vi "POP_Monitor Events.vi"() -> ()   [LabVIEW 2016]
uses:
  Ctrls/POP_Monitor Register Data.ctl
  Ctrls/POP_Event Enum.ctl
  Ctrls/POP_Popup Operation.ctl
  <vilib>/event_ctls.llb/eventvkey.ctl
  <vilib>/Utility/miscctls.llb/LVPointTypeDef.ctl
panel:
  in  "Unregister\nAll Events":bool=TRUE
  in  "Quit":refnum<user-event>
  in  "Register":refnum<user-event>
  in  "Popup":refnum<vi>
  out "error out":errorcluster
  in  "error in (no error)":errorcluster
  in  "Debug":bool
  in  "Name":string
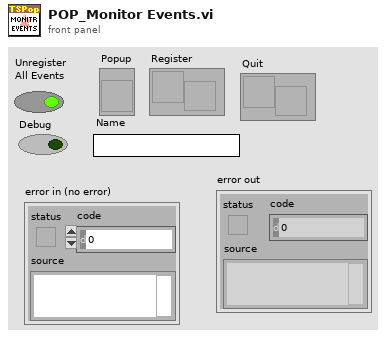
[diagram p1: front panel]
types:
  T1 = typedef "POP_Event Enum.ctl" = enum16{"Nothing", "Enter Key Accept", "Escape Key Cancel", "Mouse Outside Accept", "Mouse Outside Cancel", "Mouse Move Accept", "Mouse Move Cancel", "Mouse Leave Cancel", "Value Change Accept", "Lose Focus Cancel", "Cancel Button", "Accept Button", "Shift Ctrl Key Down"}
  T2 = typedef "eventvkey.ctl" = enum16{"ASCII", "Enter", "Return", "Shift", "Ctrl", "Alt", "Cmd", "Opt", "Caps", "NumLock", "Clear", "Break", "Up", "Down", "Left", "Right", "Insert", "Delete", "Home", "End", "PageUp", "PageDown", "Escape", "Help", "Pause", "ScrollLock", "F1", "F2", "F3", "F4", "F5", "F6", "F7", "F8", "F9", "F10", "F11", "F12", "F13", "F14", "F15", "F16", "F17", "F18", "F19", "F20", "F21", "F22", "F23", "F24", "Play", "VolumeUp", "VolumeDown", "Mute", "Two Byte Char"}
  T3 = enum32{"Bad", "Idle", "Run top level", "Running"}
  T4 = typedef "POP_Popup Operation.ctl" = enum16{"Show", "Initialize", "Close", "Popup Done", "Register a Location's Type", "Retrieve Location's Type"}
  T5 = cluster{"Shift":bool, "Ctrl":bool, "Alt":bool, "Cmd":bool, "Opt":bool}
  T6 = typedef "LVMenuShortCut.ctl" = cluster{"Include Shift Key?":bool, "Include Ctrl Key?":bool, "Shortcut Key":string}
  T7 = typedef "LVPointTypeDef.ctl" = cluster{"Horizontal":i16, "Vertical":i16}
  T8 = typedef "LVPoint32TypeDef.ctl" = cluster{"Horizontal":i32, "Vertical":i32}
  T9 = typedef "LVRectTypeDef.ctl" = cluster{"Left":i16, "Top":i16, "Right":i16, "Bottom":i16}
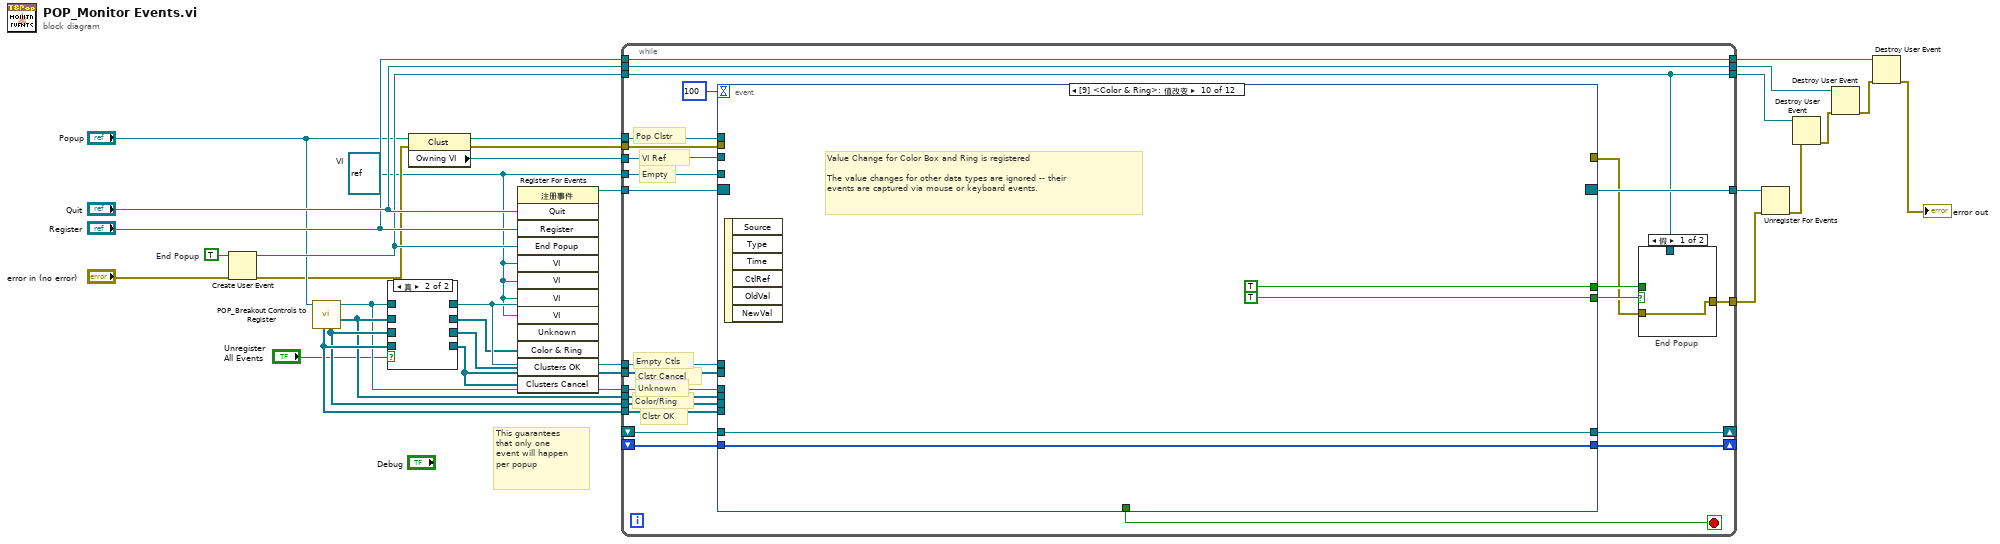
[diagram p0: block diagram]
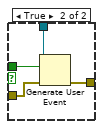
[diagram p3: hidden frame]
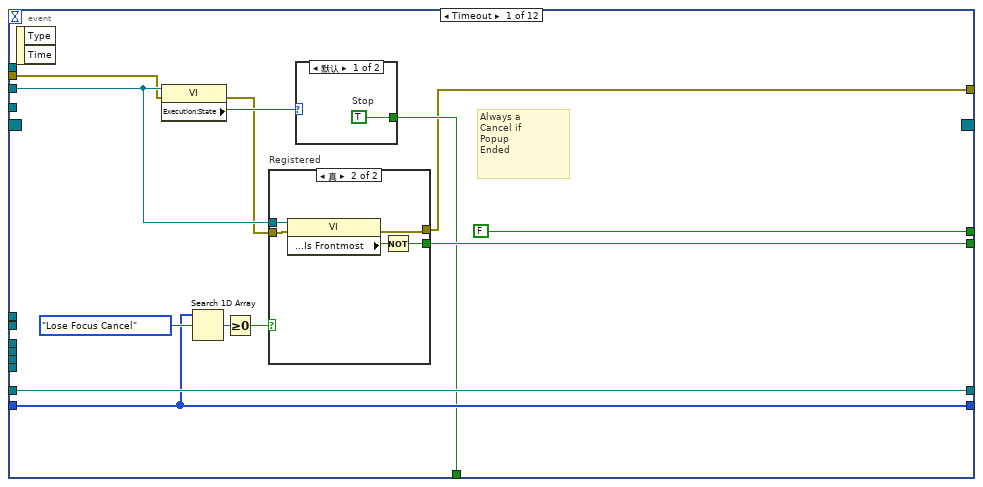
[diagram p4: hidden frame]
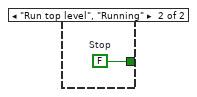
[diagram p5: hidden frame]
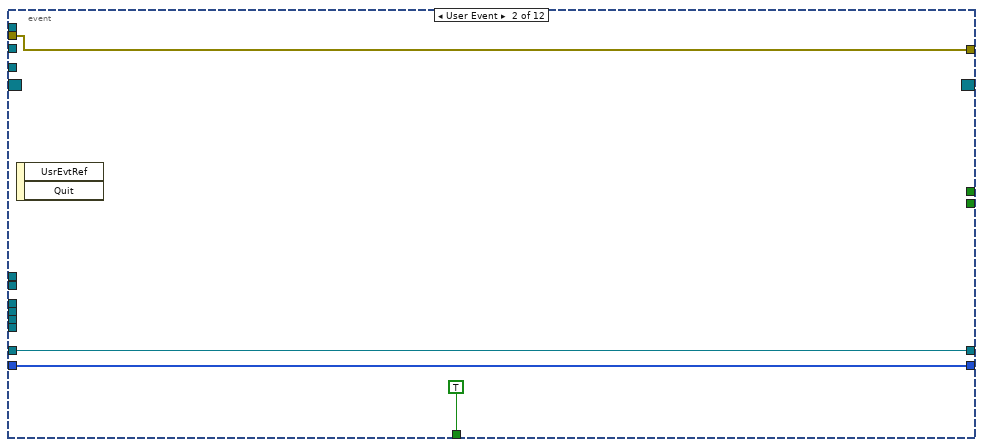
[diagram p7: hidden frame]
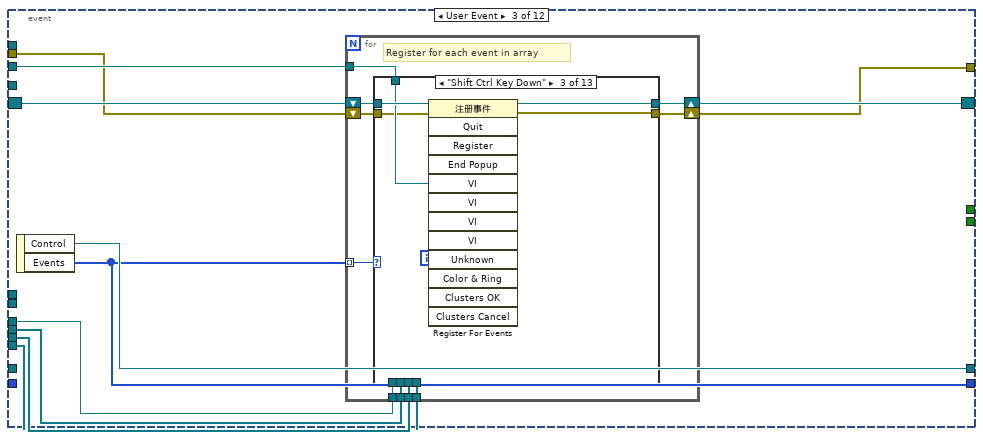
[diagram p8: hidden frame]
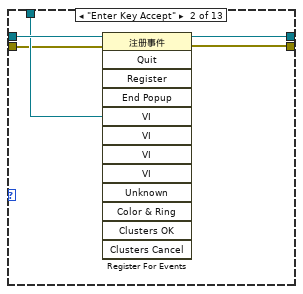
[diagram p10: hidden frame]
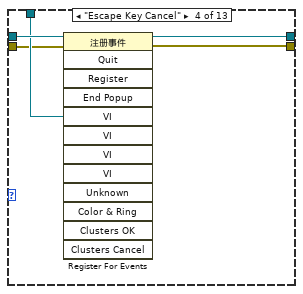
[diagram p11: hidden frame]
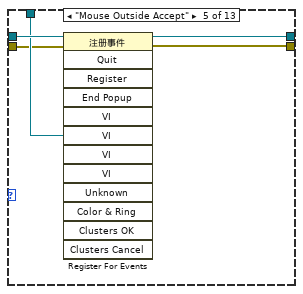
[diagram p12: hidden frame]
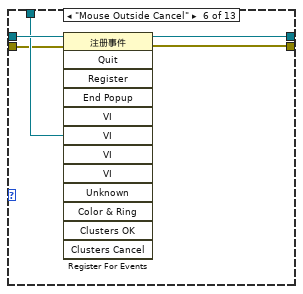
[diagram p13: hidden frame]
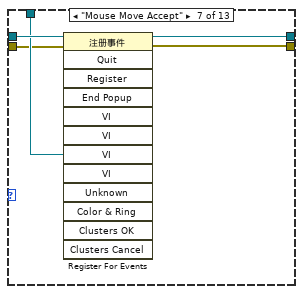
[diagram p14: hidden frame]
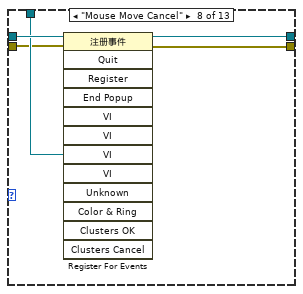
[diagram p15: hidden frame]
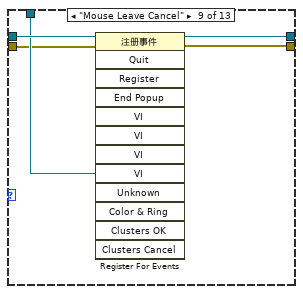
[diagram p16: hidden frame]
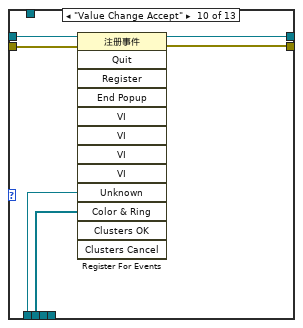
[diagram p17: hidden frame]
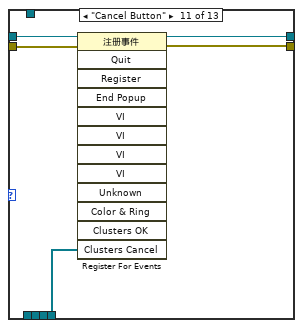
[diagram p18: hidden frame]
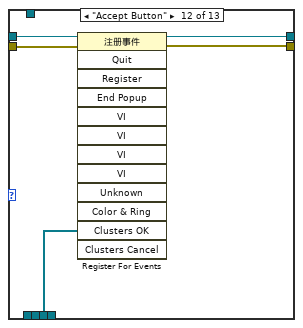
[diagram p19: hidden frame]
diagram:
  w7 = TRUE  # End Popup
  w2 = refnum<vi> refnum  # VI
  # "This guarantees\nthat only one\nevent will happen\nper popup"
  n1 = Create User Event(user event datatype=w7, error in="error in (no error)") -> (user event=w23:refnum<user-event>, error out=w3:errorcluster)
  n2 = call "POP_Breakout Controls to Register.vi"("Popup"="Popup") -> ("Color & Ring"=w19:refnum<vi>[], "Unknown"=w18:refnum<vi>, "Clusters OK"=w20:refnum<vi>[], "Clusters Cancel"=w21:refnum<vi>[])  [unwired: 7 in]
  n3 = case shown="真" "Unregister\nAll Events" {
    tunnel: [w31 _] -> w17
    tunnel: [w32 _] -> w4
    tunnel: [w33 _] -> w5
    tunnel: [w34 _] -> w16
    tunnel: w18 -> [w34 _]
    tunnel: w19 -> [w33 _]
    tunnel: w20 -> [w32 _]
    tunnel: w21 -> [w31 _]
    frame False {
    }
    frame True {
    }
  }
  n4 = property class="Clust"(reference="Popup", error in=w3) -> (reference out=w28:refnum<vi>, error out=w14:errorcluster, "Owning VI"=w1:refnum<vi>)
  n5 = register-events("Quit", "Register", w23, w2, w2, w2, w2, w16, w5, w4, w17) -> (reference out=w30:refnum<event-registration>)  [unwired: 2 in, 1 out]
  n6 = while {
    tunnel: w30 -> [w58]
    tunnel: w1 -> [w57]
    tunnel: w2 -> [w56]
    tunnel: [w55] -> w29
    tunnel: w28 -> [w54]
    tunnel: "Quit" -> [w52]
    tunnel: "Register" -> [w51]
    tunnel: [w52] -> w26
    tunnel: [w51] -> w27
    shift-right: [w50] -> _
    shift-left: _ -> [w49]
    shift-right: [w48] -> _
    shift-left: _ -> [w47]
    tunnel: w23 -> [w46]
    tunnel: [w46] -> w22
    tunnel: w21 -> [w43]
    tunnel: w20 -> [w42]
    tunnel: w19 -> [w41]
    tunnel: w18 -> [w40]
    tunnel: w17 -> [w39]
    tunnel: w16 -> [w38]
    tunnel: w14 -> [w37]
    tunnel: [w35] -> w13
    stop <- w53 stop-if-true
    # "Empty Ctls"
    # "Clstr Cancel"
    # "Clstr OK"
    # "Color/Ring"
    # "Unknown"
    # "Pop Clstr"
    # "VI Ref"
    # "Empty"
    n7 = event shown="[9] <Color & Ring>: 值改变" {
      selector: w58 -> [_ _ w99 w183 _ _ _ _ _ _ _ _]
      dyn-events: [_ _ w97 w181 _ _ _ _ _ _ _ _] -> w55
      timeout: 100 -> [_ _ _ _ _ _ _ _ _ _ _ _]
      tunnel: w57 -> [w70 _ w96 _ _ _ _ _ _ _ _ _]
      tunnel: w56 -> [_ _ _ w182 _ _ _ _ _ _ _ _]
      tunnel: w54 -> [_ _ _ _ _ w254 _ _ _ _ _ _]
      tunnel: [w68 TRUE _ _ _ _ _ _ _ _ _ _] -> w53
      tunnel: [w74 w88 w98 w185 w194 w259 w262 w270 w274 w278 w282 w286] -> w50
      tunnel: w49 -> [w74 w88 _ _ w194 w259 w262 w270 w274 w278 w282 w286]
      tunnel: [w77 w87 w100 w184 w192 w252 w266 w269 w273 w277 w281 w285] -> w48
      tunnel: w47 -> [w77 w87 _ w178 w192 w252 w266 w269 w273 w277 w281 w285]
      tunnel: [w72 _ _ _ w186 w256 TRUE TRUE TRUE TRUE TRUE TRUE] -> w45
      tunnel: [FALSE _ _ _ w187 w255 w261 FALSE FALSE TRUE TRUE FALSE] -> w44
      tunnel: w43 -> [_ _ w92 _ _ _ _ _ _ _ _ _]
      tunnel: w42 -> [_ _ w93 _ _ _ _ _ _ _ _ _]
      tunnel: w41 -> [_ _ w94 _ _ _ _ _ _ _ _ _]
      tunnel: w40 -> [_ _ w95 _ _ _ _ _ _ _ _ _]
      tunnel: w39 -> [_ _ _ w177 _ _ _ _ _ _ _ _]
      tunnel: w38 -> [_ _ _ w176 _ _ _ _ _ _ _ _]
      tunnel: w37 -> [w67 w86 w91 w175 _ w253 _ _ _ _ _ _]
      tunnel: [w65 w86 w90 w172 _ w241 _ _ _ _ _ _] -> w36
      event Timeout {
        # "Always a\nCancel if\nPopup\nEnded"
        n8 = event-data() -> ()  [unwired: 1 in, 2 out]
        n9 = property class="VI"(reference=w70, error in=w67) -> (error out=w66:errorcluster, "Execution:State"=w69:T3)  [unwired: 1 out]
        n10 = Search 1D Array(1D array=w74, element=POP_Event_Enum."Lose Focus Cancel" ("Registered Events")) -> (index of element=w76:i32)  [unwired: 1 in]
        n11 = Greater Or Equal To 0?(x=w76) -> (x >= 0?=w73:bool)
        n12 = case "Registered" shown="真" w73 {
          tunnel: w70 -> [_ w83]
          tunnel: [_ w84] -> w72
          tunnel: w66 -> [w80 w82]
          tunnel: [w80 w81] -> w65
          frame False {
          }
          frame True {
            n13 = property class="VI"(reference=w83, error in=w82) -> (error out=w81:errorcluster, "Front Panel Window:Is Frontmost"=w85:bool)  [unwired: 1 out]
            n14 = Not(x=w85) -> (.not. x?=w84:bool)
          }
        }
        n15 = case shown="默认" w69 {
          tunnel: [w78 w79] -> w68
          frame Default {
            w78 = TRUE  # Stop
          }
          frame "Run top level", "Running" {
            w79 = FALSE  # Stop
          }
        }
      }
      event User Event {
        n16 = event-data() -> ()  [unwired: 1 in, 2 out]
      }
      event User Event {
        n17 = event-data() -> ("Control"=w100:refnum<vi>, "Events"=w98:T1[])  [unwired: 1 in]
        n18 = for {
          shift-right: [w108] -> w97
          shift-left: w99 -> [w109]
          tunnel: w98 -> [w110] mode=indexing
          tunnel: w96 -> [w107]
          tunnel: w95 -> [w103]
          tunnel: w94 -> [w106]
          tunnel: w93 -> [w104]
          tunnel: w92 -> [w105]
          shift-right: [w101] -> w90
          shift-left: w91 -> [w102]
          # "Register for each event in array"
          n19 = case shown="\"Shift Ctrl Key Down\"" w110 {
            tunnel: w109 -> [w112 w117 w122 w126 w132 w137 w142 w147 w152 w158 w163 w168 w170]
            tunnel: [w112 w116 w121 w127 w131 w136 w141 w146 w151 w157 w162 w167 w170] -> w108
            tunnel: w107 -> [_ w115 w120 w125 w130 w135 w140 w145 w150 _ _ _ _]
            tunnel: w106 -> [_ _ _ _ _ _ _ _ _ w156 _ _ _]
            tunnel: w105 -> [_ _ _ _ _ _ _ _ _ _ w161 _ _]
            tunnel: w104 -> [_ _ _ _ _ _ _ _ _ _ _ w166 _]
            tunnel: w103 -> [_ _ _ _ _ _ _ _ _ w155 _ _ _]
            tunnel: w102 -> [w111 w114 w119 w124 w129 w134 w139 w144 w149 w154 w160 w165 w169]
            tunnel: [w111 w113 w118 w123 w128 w133 w138 w143 w148 w153 w159 w164 w169] -> w101
            frame "Nothing" {
              # "Nothing to register, this\nis default enum value"
            }
            frame "Enter Key Accept" {
              n20 = register-events(reference=w117, error in=w114, w115) -> (reference out=w116:refnum<event-registration>, error out=w113:errorcluster)  [unwired: 10 in]
            }
            frame "Shift Ctrl Key Down" {
              n21 = register-events(reference=w122, error in=w119, w120) -> (reference out=w121:refnum<event-registration>, error out=w118:errorcluster)  [unwired: 10 in]
            }
            frame "Escape Key Cancel" {
              n22 = register-events(reference=w126, error in=w124, w125) -> (reference out=w127:refnum<event-registration>, error out=w123:errorcluster)  [unwired: 10 in]
            }
            frame "Mouse Outside Accept" {
              n23 = register-events(reference=w132, error in=w129, w130) -> (reference out=w131:refnum<event-registration>, error out=w128:errorcluster)  [unwired: 10 in]
            }
            frame "Mouse Outside Cancel" {
              n24 = register-events(reference=w137, error in=w134, w135) -> (reference out=w136:refnum<event-registration>, error out=w133:errorcluster)  [unwired: 10 in]
            }
            frame "Mouse Move Accept" {
              n25 = register-events(reference=w142, error in=w139, w140) -> (reference out=w141:refnum<event-registration>, error out=w138:errorcluster)  [unwired: 10 in]
            }
            frame "Mouse Move Cancel" {
              n26 = register-events(reference=w147, error in=w144, w145) -> (reference out=w146:refnum<event-registration>, error out=w143:errorcluster)  [unwired: 10 in]
            }
            frame "Mouse Leave Cancel" {
              n27 = register-events(reference=w152, error in=w149, w150) -> (reference out=w151:refnum<event-registration>, error out=w148:errorcluster)  [unwired: 10 in]
            }
            frame "Value Change Accept" {
              n28 = register-events(reference=w158, error in=w154, w155, w156) -> (reference out=w157:refnum<event-registration>, error out=w153:errorcluster)  [unwired: 9 in]
            }
            frame "Cancel Button" {
              n29 = register-events(reference=w163, error in=w160, w161) -> (reference out=w162:refnum<event-registration>, error out=w159:errorcluster)  [unwired: 10 in]
            }
            frame "Accept Button" {
              n30 = register-events(reference=w168, error in=w165, w166) -> (reference out=w167:refnum<event-registration>, error out=w164:errorcluster)  [unwired: 10 in]
            }
            frame "Lose Focus Cancel" {
              # "NOOP - checked in Timeout case"
            }
          }
        }
      }
      event User Event {
        w180 = POP_Popup_Operation."Popup Done"  # Popup Operation
        w184 = refnum<vi> refnum  # Control
        w185 = T1[] [] items=["Nothing", "Enter Key Accept", "Escape Key Cancel", "Mouse Outside Accept", "Mouse Outside Cancel", "Mouse Move Accept", "Mouse Move Cancel", "Mouse Leave Cancel", "Value Change Accept", "Lose Focus Cancel", "Cancel Button", "Accept Button", "Shift Ctrl Key Down"]  # Events
        n31 = event-data() -> ("End Popup"=w179:bool)  [unwired: 1 in]
        n32 = register-events(reference=w183, error in=w175, w182, w182, w182, w182, w176, w177, w177, w177) -> (reference out=w181:refnum<event-registration>, error out=w174:errorcluster)  [unwired: 3 in]
        n33 = call "POP_FG.Popup.vi"("Popup Operation"=w180, "Name"="Name", "Error In"=w174, "Popup Accepted?"=w179) -> ("Error Out"=w173:errorcluster)  [unwired: 8 in, 3 out]
        n34 = Close Reference(reference=w178, error in (no error)=w173) -> (error out=w172:errorcluster)
      }
      event Key Down? {
        w201 = POP_Event_Enum."Escape Key Cancel"  # element
        # "Enter = Accept Popup"
        # "Registered Key Pressed"
        # "Check that key is \nRegistered and Pressed"
        # "Verify that\nkey was also\nregistered"
        # "Check if correct\nkey was pressed"
        n35 = event-data() -> ("VKey"=w190:T2, "FocusObj"=w193:refnum<vi>, "Char"=w191:i16, "PlatMods"=w189:T5)  [unwired: 1 in]
        n36 = call <vilib>:"compatReturnToEnter.vi"("VKey"=w190) -> ("VKey"=w206:T2)
        n37 = Search 1D Array(1D array=w194, element=w201) -> (index of element=w200:i32)  [unwired: 1 in]
        n38 = Search 1D Array(1D array=w194, element=POP_Event_Enum."Enter Key Accept") -> (index of element=w204:i32)  [unwired: 1 in]
        n39 = Search 1D Array(1D array=w194, element=POP_Event_Enum."Shift Ctrl Key Down" ("元素")) -> (index of element=w207:i32)  [unwired: 1 in]
        n40 = Greater Or Equal To 0?(x=w200) -> (x >= 0?=w202:bool)
        n41 = Greater Or Equal To 0?(x=w204) -> (x >= 0?=w205:bool)
        n42 = Greater Or Equal To 0?(x=w207) -> (x >= 0?=w209:bool)
        n43 = case shown="真" w209 {
          tunnel: w193 -> [_ w217]
          tunnel: w191 -> [_ w216]
          tunnel: w190 -> [_ w215]
          tunnel: w189 -> [_ w214]
          tunnel: [_ w213] -> w210
          frame False {
          }
          frame True {
            n44 = property class="GObj"(reference=w217) -> (reference out=w211:refnum<vi>, "ClassID"=w212:u32)  [unwired: 1 in, 1 out]
            n45 = case shown="27" w212 {
              tunnel: w211 -> [_ w228]
              tunnel: w216 -> [_ w221]
              tunnel: w215 -> [_ w220]
              tunnel: w214 -> [_ w219]
              tunnel: [_ w218] -> w213
              frame Default {
              }
              frame 27 {
                w227 = refnum<vi> refnum  # 字符串
                n46 = To More Specific Class(target class=w227, reference=w228) -> (specific class reference=w222:refnum<vi>)  [unwired: 1 in, 1 out]
                n47 = call "MENU_Shortcut Generate.vi"("PlatMods"=w219, "VKey"=w220, "Char"=w221) -> ("short cut"=w223:T6)  [unwired: 8 in]
                n48 = Unbundle(w223) -> ("Include Shift Key?"=w224:bool, "Include Ctrl Key?"=w225:bool, "Shortcut Key"=w226:string)
                n49 = case shown="\"True\", 默认" w226 {
                  selector: w226 -> [_ w232]
                  tunnel: w224 -> [_ w236]
                  tunnel: w225 -> [_ w235]
                  tunnel: w222 -> [_ w233]
                  tunnel: [_ TRUE] -> w218
                  frame " " {
                  }
                  frame "True", Default {
                    w237 = "" ("f")
                    # "字符串键按下"
                    n50 = Select(t="Shift+", s=w236, f=w237) -> (s? t:f=w231:string)
                    n51 = Select(t="Ctrl+", s=w235, f=w237) -> (s? t:f=w230:string)
                    n52 = Concatenate Strings(w230, w231, w232) -> (w234:string)
                    n53 = property class="Str"(reference=w233, "Value"=w234) -> ()  [unwired: 1 in, 2 out]
                  }
                }
              }
            }
          }
        }
        n54 = Equal?(x=eventvkey."Escape" ("VKey"), y=w206) -> (x = y?=w197:bool)
        n55 = Equal?(x=w206, y=eventvkey."Enter") -> (x = y?=w199:bool)
        n56 = And(x=w197, y=w202) -> (x .and. y?=w198:bool)
        n57 = And(x=w205, y=w199) -> (x .and. y?=w187:bool)
        n58 = Compound Arithmetic op=OR(w198, w187) -> (w186:bool)
        n59 = Compound Arithmetic op=OR(w186, w210) -> (w188:bool)
        n60 = event-data("Discard?"=w188) -> ()  [unwired: 1 in, 1 out]
      }
      event Mouse Down? {
        (unwired) T7 {"Horizontal"=0, "Vertical"=0} ("Pane Coordinates")
        # ">> Notes: 此处50为经验值；2014.7.30<<"
        n61 = event-data() -> ("Coords"=w240:T8)  [unwired: 1 in]
        n62 = call "POP_CtlRect.vi"("Error In"=w253, "CtlRef"=w252, "PopupRef"=w254) -> ("Error Out"=w242:errorcluster, "Panes?"=w247:bool, "Pane Refnum"=w251:refnum<vi>)  [unwired: 5 in, 1 out]
        n63 = invoke class="Pane" method="CvtPanelToPaneCoords"(reference=w251, error in=w242, "PanelCoords"=w240) -> (error out=w241:errorcluster, "PaneCoords"=w246:T7)  [unwired: 2 in, 3 out]
        n64 = Add(x=w246, y=i16 50) -> (x+y=w245:T7)
        n65 = property class="Ctl"(reference=w252) -> ("Total Bounds Rect"=w249:T9)  [unwired: 1 in, 2 out]
        n66 = Select(t=w240, s=w247, f=w245) -> (s? t:f=w244:T8)
        n67 = To Double Precision Float(number=w244) -> (double precision float=w243:cluster{"Horizontal":dbl, "Vertical":dbl})
        n68 = To Word Integer(number=w249) -> (16bit integer=w248:T9)
        n69 = call <vilib>:"PointInRect.vi"("rect"=w248, "point"=w243) -> ("pt in rect"=w257:bool)
        n70 = Not(x=w257) -> (.not. x?=w256:bool)
        n71 = Search 1D Array(1D array=w259, element=POP_Event_Enum."Mouse Outside Accept" ("Registered Events")) -> (index of element=w260:i32)  [unwired: 1 in]
        n72 = Greater Or Equal To 0?(x=w260) -> (x >= 0?=w255:bool)
        n73 = event-data("Discard?"=w256) -> ()  [unwired: 1 in, 1 out]
      }
      event Mouse Move {
        # "Used for Rings to capture when the selection doesn't change\nand for both rings and colorboxes when Escape is pressed \n(not captured with Key Press event)"
        n74 = event-data() -> ()  [unwired: 1 in, 1 out]
        n75 = Search 1D Array(1D array=w262, element=POP_Event_Enum."Mouse Move Accept" ("Registered Events")) -> (index of element=w264:i32)  [unwired: 1 in]
        n76 = Greater Or Equal To 0?(x=w264) -> (x >= 0?=w261:bool)
      }
      event Mouse Leave {
        # "Mouse Leave is (currently) always registered as a cancel.\nThis is used for Colors and Rings to capture when the Escape key is\npressed when the mouse is outside the window."
        n77 = event-data() -> ()  [unwired: 1 in, 1 out]
      }
      event Value Change {
        # "If Data Type is unknown, a Button is displayed.\n\nReturn Canceled after button is pressed"
        n78 = event-data() -> ()  [unwired: 1 in, 6 out]
      }
      event Value Change {
        # "Value Change for Color Box and Ring is registered\n\nThe value changes for other data types are ignored -- their\nevents are captured via mouse or keyboard events."
        n79 = event-data() -> ()  [unwired: 1 in, 6 out]
      }
      event Value Change {
        n80 = event-data() -> ()  [unwired: 1 in, 6 out]
      }
      event Value Change {
        n81 = event-data() -> ()  [unwired: 1 in, 6 out]
      }
    }
    n82 = case "End Popup" shown="假" w45 {
      tunnel: w46 -> [_ w64]
      tunnel: w44 -> [_ w63]
      tunnel: w36 -> [w60 w62]
      tunnel: [w60 w61] -> w35
      frame False {
      }
      frame True {
        n83 = Generate User Event(user event=w64, event data cluster=w63, error in=w62) -> (error out=w61:errorcluster)  [unwired: 1 in, 1 out]
      }
    }
  }
  n84 = Unregister For Events(event registration refnum=w29, error in=w13) -> (error out=w12:errorcluster)
  n85 = Destroy User Event(user event=w22, error in=w12) -> (error out=w11:errorcluster)
  n86 = Destroy User Event(user event=w26, error in=w11) -> (error out=w10:errorcluster)
  n87 = Destroy User Event(user event=w27, error in=w10) -> (error out=→"error out":errorcluster)
